vi "自动添加所有参数数据.vi"(8 "error in (no error)":errorcluster, 11 "数据类别":enum16{"水样数据", "日质控数据"}(ring)) -> (0 "错误输出":errorcluster)   [LabVIEW 2016, in "数据查询.lvlib"]
uses:
  <vilib>/Utility/sysdir.llb/System Directory Type.ctl
  <vilib>/addons/database/Connection.llb/DB Tools Open Connec (String).vi
  <vilib>/Utility/config.llb/Read Key (String).vi
  <vilib>/Utility/config.llb/Write Key (String).vi
  <vilib>/addons/database/NI_Database_API.lvlib
  <vilib>/Utility/config.llb/NI_LVConfig.lvlib
panel:
  out "数组":timestamp[](array[timestamp])
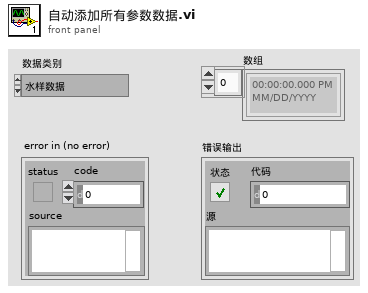
[diagram p1: front panel]
types:
  T1 = typedef "System Directory Type.ctl" = i32
  T2 = typedef "NI_Database_API.lvlib/Conn ObjectReference.ctl" = refnum<k1>
  T3 = typedef "NI_LVConfig.lvlib/Config Data RefNum.ctl" = refnum<k1>
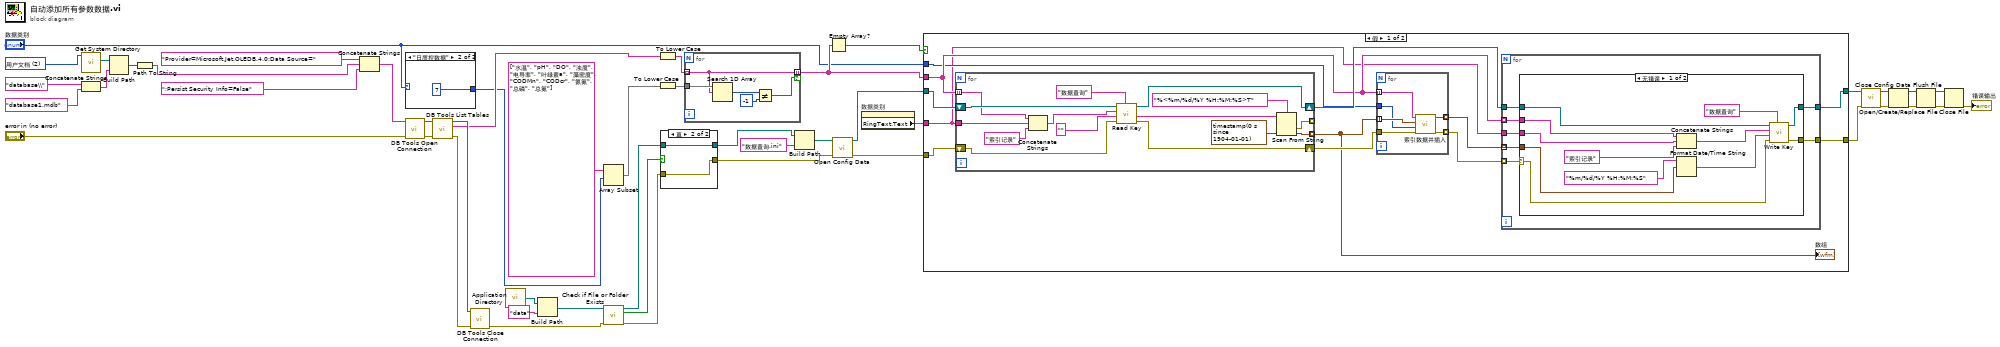
[diagram p0: block diagram]
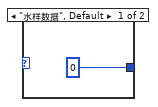
[diagram p2: hidden frame]
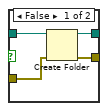
[diagram p5: hidden frame]
diagram:
  w47 = T1 2 items=["用户目录"=0, "用户桌面"=1, "用户文档"=2, "用户应用程序数据"=3, "用户设置"=4, "用户临时目录"=5, "公共文档"=6, "公共应用程序数据"=7, "公共设置"=8, "公共缓存"=13, "系统核心库"=9, "系统安装库"=10, "应用程序文件"=11, "启动盘根目录"=12] ("system directory type")
  n1 = call <vilib>:"Get System Directory.vi"("system directory type"=w47) -> ("system directory"=w45:path)  [unwired: 10 in]
  n2 = Concatenate Strings("database\\" ("condition"), "database1.mdb" ("字符串")) -> (w39:string)
  n3 = Build Path(base path=w45, name or relative path=w39) -> (appended path=w44:path)
  n4 = Path To String(path=w44) -> (string=w43:string)
  n5 = Concatenate Strings("Provider=Microsoft.Jet.OLEDB.4.0;Data Source=" ("condition"), w43, ";Persist Security Info=False" ("condition")) -> (w41:string)
  n6 = case shown="\"日质控数据\"" "数据类别" {
    tunnel: [0 7] -> w2
    frame "水样数据", Default {
    }
    frame "日质控数据" {
    }
  }
  n7 = call-poly <vilib>:"DB Tools Open Connection.vi"("error in (no error)"="error in (no error)", "connection information"=w41) -> ("error out"=w35:errorcluster, "connection reference"=w36:T2)  [unwired: 6 in]
  n8 = call <vilib>:"DB Tools List Tables.vi"("error in (no error)"=w35, "connection reference"=w36) -> ("error out"=w34:errorcluster, "tables"=w31:string[], "connection reference out"=w33:T2)  [unwired: 3 in]
  n9 = call <vilib>:"DB Tools Close Connection.vi"("error in (no error)"=w34, "connection reference"=w33) -> ("error out"=w6:errorcluster)  [unwired: 5 in]
  n10 = call <vilib>:"Application Directory.vi"() -> ("Application Directory"=w22:path)
  n11 = Build Path(base path=w22, name or relative path="data" ("名称或相对路径")) -> (appended path=w24:path)
  n12 = Array Subset(array=string[] ["水温", "pH", "DO", "浊度", "电导率", "叶绿素a", "藻密度", "CODMn", "CODcr", "氨氮", "总磷", "总氮"], index=w2) -> (w1:string[])  [unwired: 1 in]
  n13 = call <vilib>:"Check if File or Folder Exists.vi"("error in (no error)"=w6, "path"=w24) -> ("error out"=w27:errorcluster, "file or folder exists?"=w25:bool, "dup path"=w26:path)  [unwired: 7 in]
  n14 = To Lower Case(string=w31) -> (all lower case string=w30:string[])
  n15 = To Lower Case(string=w1) -> (all lower case string=w32:string[])
  n16 = case shown="真" w25 {
    tunnel: w26 -> [w53 w55]
    tunnel: w27 -> [w52 w54]
    tunnel: [w51 w55] -> w28
    tunnel: [w50 w54] -> w13
    frame False {
      n17 = Create Folder(path (use dialog)=w53, error in=w52) -> (created path=w51:path, error out=w50:errorcluster)  [unwired: 1 in, 1 out]
    }
    frame True {
    }
  }
  n18 = for {
    tunnel: w30 -> [w57] mode=indexing
    tunnel: w32 -> [w60]
    tunnel: [w57] -> w10 mode=indexing if=w56
    n19 = Search 1D Array(1D array=w60, element=w57) -> (index of element=w59:i32)  [unwired: 1 in]
    n20 = Not Equal?(x=w59, y=-1) -> (x != y?=w56:bool)
  }
  n21 = Build Path(base path=w28, name or relative path="数据查询.ini" ("名称或相对路径")) -> (appended path=w21:path)
  n22 = Empty Array?(array=w10) -> (empty?=w9:bool)
  n23 = call <vilib>:"Open Config Data.vi"("error in (no error)"=w13, "configuration file path"=w21) -> ("error out"=w11:errorcluster, "refnum"=w12:T3)  [unwired: 7 in, 1 out]
  n24 = property on="数据类别" class="Enum (严格)"() -> ("RingText.Text"=w7:string)  [unwired: 2 in, 2 out]
  n25 = case shown="假" w9 {
    tunnel: [w71 w116] -> w15
    tunnel: [w70 w115] -> w14
    tunnel: w12 -> [w69 w116]
    tunnel: w11 -> [w68 w115]
    tunnel: w10 -> [w66 _]
    tunnel: "数据类别" -> [w63 _]
    tunnel: w7 -> [w62 _]
    frame False {
      n26 = for {
        shift-right: [w106] -> w67
        shift-left: w69 -> [w108]
        shift-right: [w105] -> w65
        shift-left: w68 -> [w107]
        tunnel: w66 -> [w97] mode=indexing
        tunnel: [w99] -> w61 mode=indexing
        tunnel: [w98] -> _ mode=indexing
        tunnel: w62 -> [w96]
        n27 = Concatenate Strings(w97, w96, "索引记录" ("key")) -> (w102:string)
        n28 = call-poly <vilib>:"Read Key.vi"("section"="数据查询", "error in (no error)"=w107, "default value"="", "key"=w102, "refnum"=w108) -> ("error out"=w105:errorcluster, "value"=w95:string, "refnum out"=w106:T3)  [unwired: 3 in, 1 out]
        n29 = Scan From String(format string="%<%m/%d/%Y %H:%M:%S>T" ("格式字符串"), input string=w95, default 1=timestamp(0 s since 1904-01-01) ("默认值 1")) -> (error out=w98:errorcluster, output 1=w99:timestamp)  [unwired: 2 in, 2 out]
      }
      "数组" <- w61
      n30 = for {
        tunnel: w61 -> [w114] mode=indexing
        tunnel: w66 -> [w113] mode=indexing
        tunnel: [w112] -> w64 mode=indexing
        tunnel: [w111] -> w72 mode=indexing
        tunnel: w65 -> [w110]
        tunnel: w63 -> [w109]
        n31 = call "索引数据并插入.vi"("error in (no error)"=w110, "数据类别"=w109, "索引记录"=w114, "table"=w113) -> ("error out"=w112:errorcluster, "最新索引记录"=w111:timestamp)  [unwired: 6 in]
      }
      n32 = for {
        tunnel: w66 -> [w79] mode=indexing
        tunnel: w72 -> [w78] mode=indexing
        tunnel: w67 -> [w77]
        tunnel: w64 -> [w74] mode=indexing
        tunnel: [w76] -> w71
        tunnel: [w75] -> w70
        tunnel: w62 -> [w73]
        n33 = case shown="无错误" w74 {
          selector: w74 -> [w82 w92]
          tunnel: w79 -> [w81 _]
          tunnel: w78 -> [w88 _]
          tunnel: w77 -> [w86 w93]
          tunnel: [w85 w93] -> w76
          tunnel: [w84 w92] -> w75
          tunnel: w73 -> [w80 _]
          frame No Error {
            n34 = Concatenate Strings(w81, w80, "索引记录" ("key")) -> (w89:string)
            n35 = Format Date/Time String(time format string (%c)="%m/%d/%Y %H:%M:%S" ("时间格式字符串(%c)"), seconds (now)=w88) -> (date/time string=w87:string)  [unwired: 1 in]
            n36 = call-poly <vilib>:"Write Key.vi"("section"="数据查询", "error in (no error)"=w82, "value"=w87, "key"=w89, "refnum"=w86) -> ("error out"=w84:errorcluster, "refnum out"=w85:T3)  [unwired: 4 in, 1 out]
          }
          frame Error {
          }
        }
      }
    }
    frame True {
    }
  }
  n37 = call <vilib>:"Close Config Data.vi"("error in (no error)"=w14, "refnum"=w15) -> ("error out"=w20:errorcluster, "file path"=w8:path)  [unwired: 8 in]
  n38 = Open/Create/Replace File(file path (use dialog)=w8, error in=w20) -> (refnum out=w16:refnum<file>, error out=w17:errorcluster)  [unwired: 4 in, 1 out]
  n39 = Flush File(refnum=w16, error in=w17) -> (refnum out=w18:refnum<file>, error out=w19:errorcluster)
  n40 = Close File(refnum=w18, error in=w19) -> (error out=→"错误输出":errorcluster)  [unwired: 1 out]
